vi "Test_logEvent_arrays.vi"(8 "error in (no error)":errorcluster, 11 "logevent_arrays_Ctl":T1={"private_rcvStamp"=0.0, "boolean0[5]"=[FALSE, FALSE, FALSE, FALSE, FALSE], "byte0[5]"=[0, 0, 0, 0, 0], "short0[5]"=[0, 0, 0, 0, 0], "int0[5]"=[0, 0, 0, 0, 0], "long0[5]"=[0, 0, 0, 0, 0], "longLong0[5]"=[0, 0, 0, 0, 0], "octet0[5]"=[0, 0, 0, 0, 0], "unsignedShort0[5]"=[0, 0, 0, 0, 0], "unsignedInt0[5]"=[0, 0, 0, 0, 0], "unsignedLong0[5]"=[0, 0, 0, 0, 0], "float0[5]"=[0.0, 0.0, 0.0, 0.0, 0.0], "double0[5]"=[0.0, 0.0, 0.0, 0.0, 0.0], "priority"=0}) -> (0 "error out":errorcluster, 2 "function return":i32, 3 "logevent_arrays_Ctl out":T1)   [LabVIEW 2018, in "SALLV_Test.lvlib"]
doc: "int Test_shm_logEvent_arraysLV(Test_logevent_arraysLV *logevent_arrays_Ctl );"
uses:
  DataTypes/logevent_arrays.ctl
  SALLV_Test.lvlib
  SALLV_Test.so
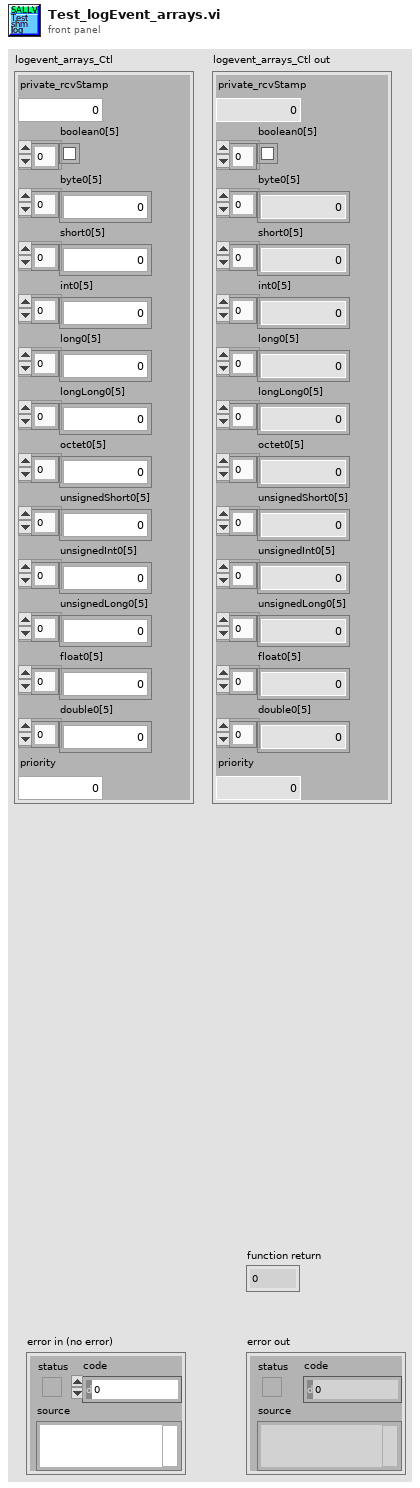
[diagram p1: front panel]
types:
  T1 = typedef "SALLV_Test.lvlib/logevent_arrays.ctl" = cluster{"private_rcvStamp":dbl, "boolean0[5]":bool[], "byte0[5]":u8[], "short0[5]":i16[], "int0[5]":i32[], "long0[5]":i32[], "longLong0[5]":i64[], "octet0[5]":u8[], "unsignedShort0[5]":u16[], "unsignedInt0[5]":u32[], "unsignedLong0[5]":u32[], "float0[5]":sgl[], "double0[5]":dbl[], "priority":i32}
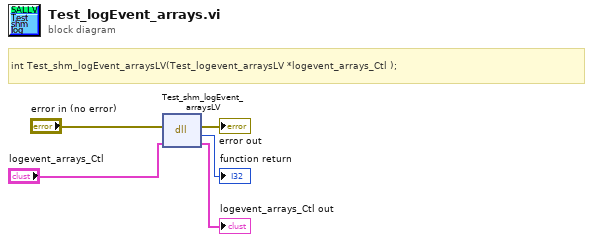
[diagram p0: block diagram]
diagram:
  # "int Test_shm_logEvent_arraysLV(Test_logevent_arraysLV *logevent_arrays_Ctl );"
  n1 = dll-call lib="home/ttsai/Documents/salTestLabViewApi/SALLV_Test/SALLV_Test.*" fn="Test_shm_logEvent_arraysLV"(error in="error in (no error)", "logevent_arrays_Ctl"="logevent_arrays_Ctl") -> (error out=→"error out":errorcluster, →"function return":i32, "logevent_arrays_Ctl"=→"logevent_arrays_Ctl out":T1)  [unwired: 2 in, 1 out]
